vi "RSZVB Set Pulse Generator Polarity.vi"(7 "Pulse Polarity (0)":i32(ring) items=["Normal", "Inverted"], 8 "error in (no error)":errorcluster {"code" format="%.0x"}, 9 "Generator (1)":i32=1, 10 "Channel (1)":i32=1, 11 "VISA session":refnum<visa-resource-name>) -> (0 "error out":errorcluster {"code" format="%.0x"}, 3 "dup VISA session":refnum<visa-resource-name>)   [LabVIEW 2011]
doc: "This VI selects the polarity of the pulse generator signal <gen_no>. \n\nNote(s):\n\n(1) This VI is available only with option R&S ZVA-K27.\n\nRemote-control command(s):\n[SENSe<Ch>:]PULSe:GENerator<gen_no>:POLarity NORMal | INVerted"
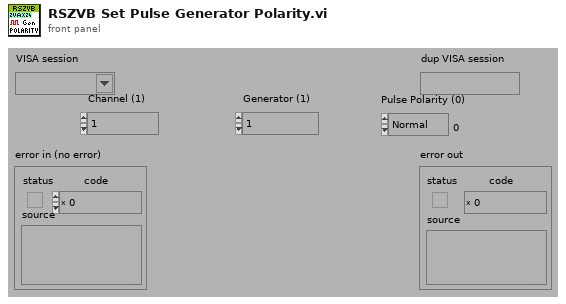
[diagram p1: front panel]
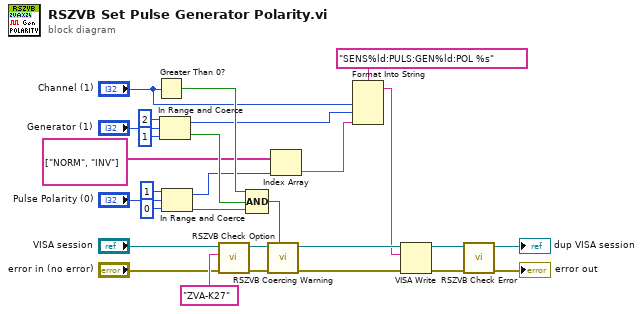
[diagram p0: block diagram]
diagram:
  n1 = Greater Than 0?(x="Channel (1)") -> (x > 0?=w12:bool)
  n2 = In Range and Coerce(upper limit=2, x="Generator (1)", lower limit=1) -> (coerced(x)=w11:i32, In Range?=w13:bool)
  n3 = In Range and Coerce(upper limit=1, x="Pulse Polarity (0)", lower limit=0) -> (coerced(x)=w10:i32, In Range?=w14:bool)
  n4 = call "RSZVB Check Option.vi"("error in (no error)"="error in (no error)", "Options"="ZVA-K27", "VISA session"="VISA session") -> ("error out"=w22:errorcluster, "dup VISA session"=w21:refnum<visa-resource-name>)  [unwired: 7 in]
  n5 = Compound Arithmetic op=AND(w12, w13, w14) -> (w16:bool)
  n6 = call "RSZVB Coercing Warning.vi"("In Range?"=w16, "error in (no error)"=w22, "VISA session"=w21) -> ("error out"=w27:errorcluster, "dup VISA session"=w28:refnum<visa-resource-name>)  [unwired: 7 in]
  n7 = Index Array(array=string[] ["NORM", "INV"], index=w10) -> (element=w9:string)
  n8 = Format Into String(format string="SENS%ld:PULS:GEN%ld:POL %s", "Channel (1)", w11, w9) -> (resulting string=w24:string)  [unwired: 2 in, 1 out]
  n9 = VISA Write(VISA resource name=w28, write buffer=w24, error in (no error)=w27) -> (VISA resource name out=w25:refnum<visa-resource-name>, error out=w26:errorcluster)  [unwired: 1 out]
  n10 = call "RSZVB Check Error.vi"("error in (no error)"=w26, "VISA session"=w25) -> ("error out"=→"error out":errorcluster, "dup VISA session"=→"dup VISA session":refnum<visa-resource-name>)  [unwired: 8 in]
